vi "Write Right Synced Motors.vi"(8 "error in (no error)":errorcluster, 10 "Actor Framework:Message Enqueuer":refnum<class "Message Enqueuer.lvclass">, 11 "Forward Drive in":refnum<class "Forward Drive.lvclass">) -> (0 "error out":errorcluster, 3 "Forward Drive out":refnum<class "Forward Drive.lvclass">)   [LabVIEW 2014, in "Forward Drive.lvlib" / "Forward Drive.lvclass"]
uses:
  Forward Drive.lvclass
  <vilib>/ActorFramework/Message Enqueuer/Message Enqueuer.lvclass
  Forward Drive.lvclass/Forward Drive.ctl
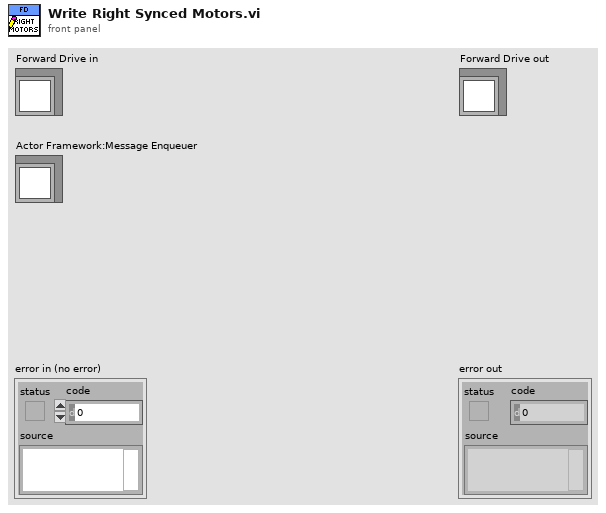
[diagram p1: front panel]
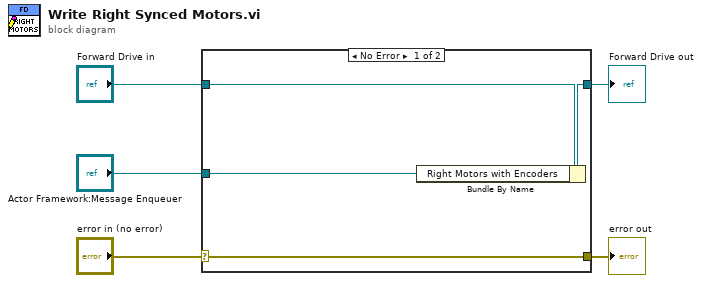
[diagram p0: block diagram]
diagram:
  n1 = case shown="No Error" "error in (no error)" {
    selector: "error in (no error)" -> [w9 w10]
    tunnel: [w9 w10] -> w4
    tunnel: [w7 w11] -> w2
    tunnel: "Forward Drive in" -> [w8 w11]
    tunnel: "Actor Framework:Message Enqueuer" -> [w6 _]
    frame No Error {
      n2 = Bundle By Name(cluster=w8, "Right Motors with Encoders"=w6) -> (w7:refnum<class "Forward Drive.lvclass">)
    }
    frame Error {
    }
  }
  "error out" <- w4
  "Forward Drive out" <- w2
